vi "Function.vi"(8 "error in (no error)":errorcluster, 10 "Waveform":waveform(dbl), 11 "Two Terminal in":refnum<class "AbsFunc_One Term_WFM_Numeric.lvclass">) -> (0 "error out":errorcluster, 2 "Result":waveform(dbl), 3 "Two Terminal out":refnum<class "AbsFunc_One Term_WFM_Numeric.lvclass">)   [LabVIEW 2021, in "AbsFunc_One Term_WFM_Numeric.lvclass"]
uses:
  AbsFunc_One Term_WFM_Numeric.lvclass
  AbsFunc_One Term_WFM_Numeric.lvclass/AbsFunc_One Term_WFM_Numeric.ctl
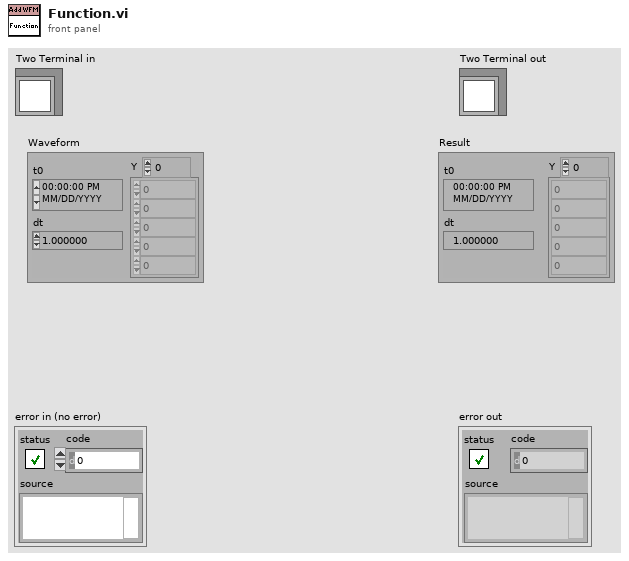
[diagram p1: front panel]
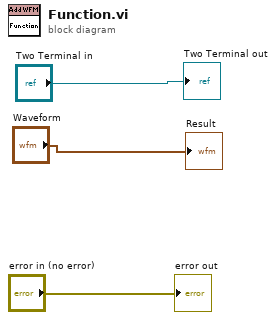
[diagram p0: block diagram]
diagram:
  "error out" <- "error in (no error)"
  "Two Terminal out" <- "Two Terminal in"
  "Result" <- "Waveform"
